vi "Lightning Begin.vi"() -> (0 "error out":errorcluster)   [LabVIEW 2014]
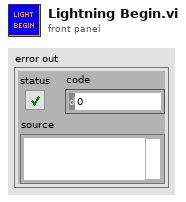
[diagram p1: front panel]
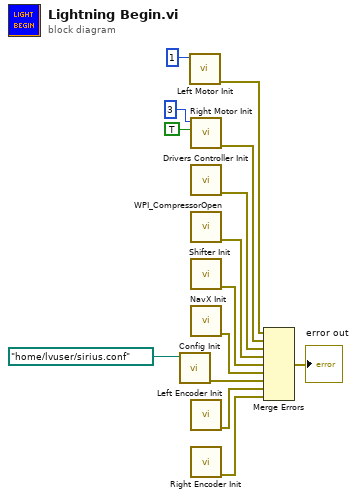
[diagram p0: block diagram]
diagram:
  n1 = call "Config Init.vi"("Path"=path "/home/lvuser/sirius.conf") -> ("error out"=w4:errorcluster)  [unwired: 10 in]
  n2 = call "Left Motor Init.vi"("CAN Id"=u8 1) -> ("error out"=w10:errorcluster)  [unwired: 10 in]
  n3 = call "Right Motor Init.vi"("Invert (default false)"=TRUE, "CAN Id"=u8 3) -> ("error out"=w11:errorcluster)  [unwired: 9 in]
  n4 = call "Drivers Controller Init.vi"() -> ("error out"=w8:errorcluster)  [unwired: 11 in]
  n5 = call <vilib>:"WPI_CompressorOpen.vi"() -> ("error out"=w7:errorcluster)  [unwired: 14 in, 1 out]
  n6 = call "Shifter Init.vi"() -> ("Error Out"=w6:errorcluster)  [unwired: 11 in]
  n7 = call "NavX Init.vi"() -> ("error out"=w5:errorcluster)  [unwired: 11 in]
  n8 = call "Left Encoder Init.vi"() -> ("error out"=w2:errorcluster)  [unwired: 11 in]
  n9 = call "Right Encoder Init.vi"() -> ("error out"=w1:errorcluster)  [unwired: 11 in]
  n10 = Merge Errors(w10, w11, w8, w7, w6, w5, w4, w2, w1) -> (→"error out":errorcluster)
